vi "onListenForNewConnection.vi"(8 "error in (no error)":errorcluster, 9 "timeout (ms)":i32=2000, 11 "Listener":refnum<class "Connection.TCP-TLS.lvclass">) -> (0 "error out":errorcluster, 1 "New connection":bool, 2 "timed out":bool, 3 "New Connection":refnum<class "Connection.lvclass">)   [LabVIEW 2020, in "Connection.TCP-TLS.lvclass"]
uses:
  Connection.TCP-TLS.lvclass
  Connection.TCP-TLS.lvclass/Connection.TCP-TLS.ctl
  <vilib>/LabVIEW Open Source Project/MQTT TCP Connection/MQTT_TCP/Connection/TCPConnection.lvclass
  C:/Program Files (x86)/National Instruments/LabVIEW 2020/vi.lib/LabVIEW Open Source Project/MQTT TCP Connection/MQTT_TCP/Connection/TCPConnection.lvclass
  C:/Program Files (x86)/National Instruments/LabVIEW 2020/vi.lib/LabVIEW Open Source Project/MQTT Connection/MQTT_Connection/Connection/Connection.lvclass
  C:/Program Files (x86)/National Instruments/LabVIEW 2020/vi.lib/LabVIEW Open Source Project/Connection/Connection/Connection.lvclass
  C:/Repositories/LVOS/MQTT-Connection-SecuredTCP/source/Connection.SecuredTCP/Connection.TCP-TLS.lvclass
  <vilib>/LabVIEW Open Source Project/Connection/Connection/Connection.lvclass
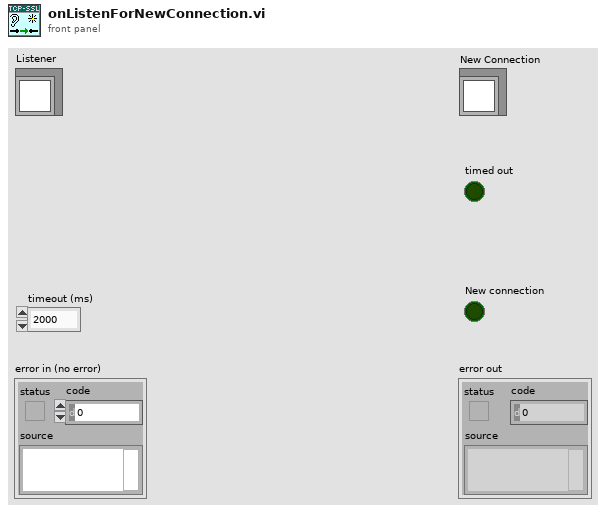
[diagram p1: front panel]
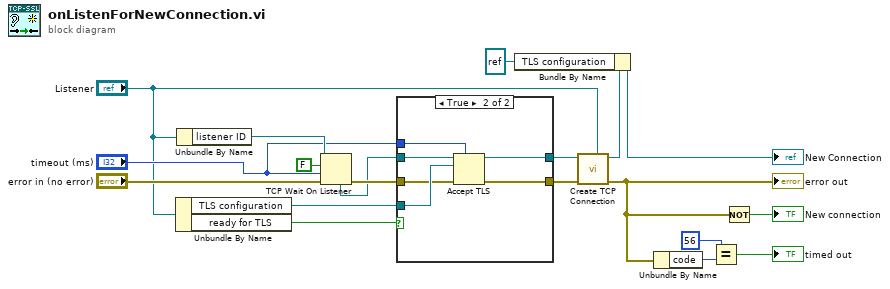
[diagram p0: block diagram]
diagram:
  n1 = Unbundle By Name("Listener") -> ("TLS configuration"=w7:refnum<k36>, "ready for TLS"=w6:bool)
  n2 = Unbundle By Name("Listener") -> ("listener ID"=w19:refnum<k5>)
  n3 = TCP Wait On Listener(8:"error in (no error)", 9:"timeout (ms)", 10:FALSE ("resolve remote address (T)"), 11:w19) -> (0:w12:errorcluster, 4:w11:refnum<k5>)  [unwired: 3 out]
  n4 = case shown="True" w6 {
    tunnel: [w21 w22] -> w3
    tunnel: w7 -> [_ w25]
    tunnel: w11 -> [w21 w27]
    tunnel: w12 -> [w20 w24]
    tunnel: [w20 w23] -> w2
    tunnel: "timeout (ms)" -> [_ w26]
    frame False {
    }
    frame True {
      n5 = Accept TLS(7:w26, 8:w24, 10:w25, 11:w27) -> (0:w23:errorcluster, 3:w22:refnum<k5>)  [unwired: 1 out]
    }
  }
  n6 = call <vilib>:"Create TCP Connection.vi"("TCPConnection in"="Listener", "error in (no error)"=w2, "connection ID"=w3) -> ("error out"=w1:errorcluster, "TCPConnection out"=w4:refnum<class "Connection.TCP-TLS.lvclass">)  [unwired: 7 in]
  "error out" <- w1
  n7 = Bundle By Name(cluster=w4, "TLS configuration"=refnum<k36> refnum) -> (→"New Connection":refnum<class "Connection.TCP-TLS.lvclass">)
  n8 = Unbundle By Name(w1) -> ("code"=w18:i32)
  n9 = Equal?(x=56, y=w18) -> (x = y?=→"timed out":bool)
  n10 = Not(x=w1) -> (.not. x?=→"New connection":bool)
